vi "Load to memory.vi"(0 "LV Doc in":refnum<class "LV Doc.lvclass">, 5 "Path":path, 11 "error in (no error)":errorcluster) -> (4 "LV Doc out":refnum<class "LV Doc.lvclass">, 15 "error out":errorcluster)   [LabVIEW 2016, in "LV Doc.lvclass"]
uses:
  LV Doc.lvclass
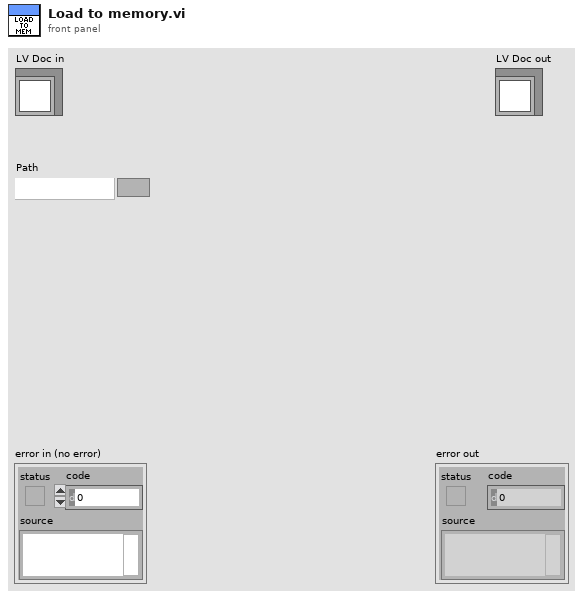
[diagram p1: front panel]
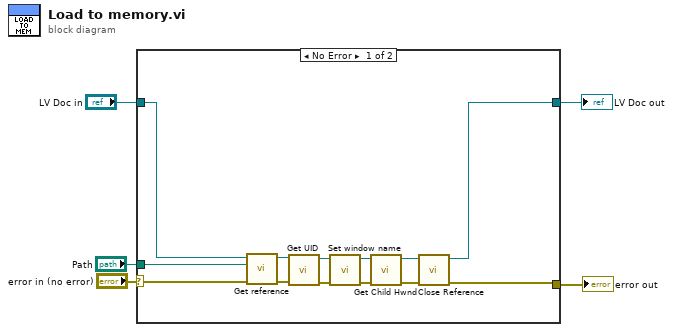
[diagram p0: block diagram]
diagram:
  n1 = case shown="No Error" "error in (no error)" {
    selector: "error in (no error)" -> [w10 w20]
    tunnel: [w11 w20] -> w4
    tunnel: "LV Doc in" -> [w9 w19]
    tunnel: [w12 w19] -> w2
    tunnel: "Path" -> [w8 _]
    frame No Error {
      n2 = call "Get reference.vi"("Error in"=w10, "Vi Path"=w8, "LV Doc.lvclass"=w9) -> ("Error Out"=w15:errorcluster, "LV Doc.lvclass"=w18:refnum<class "LV Doc.lvclass">)  [unwired: 7 in]
      n3 = call "Get UID.vi"("error in (no error)"=w15, "LV Doc.lvclass"=w18) -> ("error out"=w14:errorcluster, "LV Doc.lvclass"=w17:refnum<class "LV Doc.lvclass">)  [unwired: 8 in]
      n4 = call "Set window name.vi"("error in (no error)"=w14, "LV Doc.lvclass"=w17) -> ("error out"=w13:errorcluster, "LV Doc.lvclass"=w16:refnum<class "LV Doc.lvclass">)  [unwired: 8 in]
      n5 = call "Get Child Hwnd.vi"("Error in"=w13, "LV Doc.lvclass"=w16) -> ("Error Out"=w6:errorcluster, "LV Doc.lvclass"=w7:refnum<class "LV Doc.lvclass">)  [unwired: 8 in]
      n6 = call "Close Reference.vi"("error in (no error)"=w6, "LV Doc in"=w7) -> ("error out"=w11:errorcluster, "LV Doc out"=w12:refnum<class "LV Doc.lvclass">)  [unwired: 8 in]
    }
    frame Error {
    }
  }
  "error out" <- w4
  "LV Doc out" <- w2
